vi "Cluster.GetAllContolReferencesRecursive.vi"(6 "error in (no error)":errorcluster, 9 "cluster refnum":refnum<vi>) -> (0 "error out":errorcluster, 1 "labels[]":string[](array[string]), 2 "controls[]":refnum<vi>[](array[refnum]))   [LabVIEW 2019, in "Tools.lvlib"]
doc: "The Get All Control References VI recursively determines control references for all objects on the front panel of another VI. This VI takes a front panel reference input and returns an array of references to all controls on that front panel. This VI returns references to all elements of a cluster, including elements in embedded clusters. This VI also returns the element types of arrays embedded in cluster elements."
uses:
  Tools.lvlib
panel:
  # "Select Help»Show Context Help and move the cursor over the VI icon to display help for this VI."
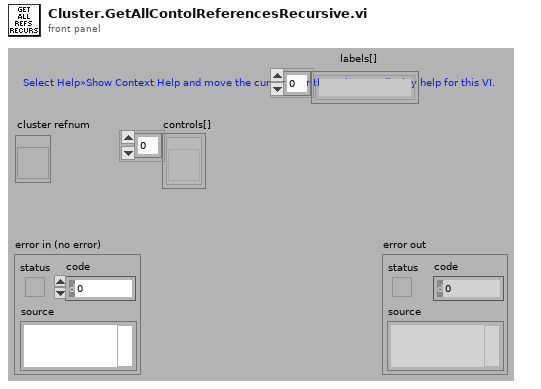
[diagram p1: front panel]
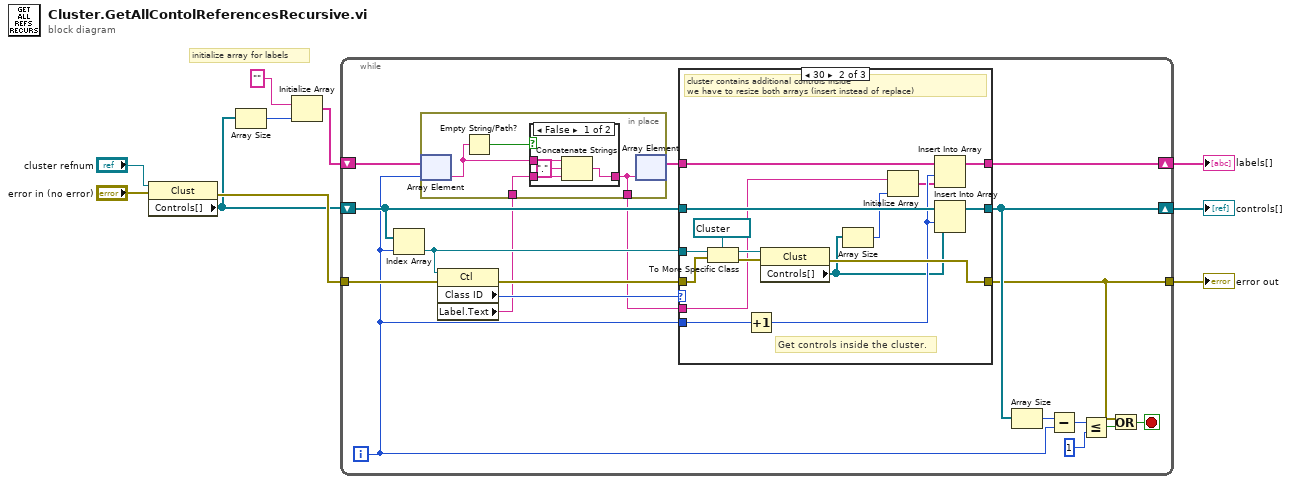
[diagram p0: block diagram]
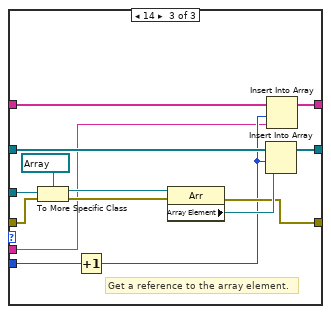
[diagram p4: hidden frame]
diagram:
  # "initialize array for labels"
  n1 = property class="Clust"(reference="cluster refnum", error in="error in (no error)") -> (error out=w8:errorcluster, "Controls[]"=w5:refnum<vi>[])  [unwired: 1 out]
  n2 = Array Size(array=w5) -> (size(s)=w4:i32)
  n3 = Initialize Array("", w4) -> (w3:string[])
  n4 = while {
    shift-right: [w20] -> w10
    shift-left: w5 -> [w21]
    tunnel: w8 -> [w19]
    tunnel: [w11] -> w7
    shift-right: [w17] -> w2
    shift-left: w3 -> [w16]
    i -> [w14]
    stop <- w24 stop-if-true
    n5 = Index Array(array=w21, index=w14) -> (element=w22:refnum<vi>)
    n6 = property class="Ctl"(reference=w22, error in=w19) -> (error out=w18:errorcluster, "Class ID"=w23:u32, "Label.Text"=w13:string)  [unwired: 1 out]
    n7 = in-place {
      in-place-border: w13 -> [w31]
      in-place-border: [w29] -> w12
      n8 = in-place-array #1(w16, w14) -> (w30:string)
      n9 = Empty String/Path?(string/path=w30) -> (empty?=w32:bool)
      n10 = case shown="False" w32 {
        tunnel: w31 -> [w35 w37]
        tunnel: [w34 w37] -> w29
        tunnel: w30 -> [w36 _]
        frame False {
          n11 = Concatenate Strings(w36, "." ("string"), w35) -> (w34:string)
        }
        frame True {
        }
      }
      n12 = in-place-array #1(w29) -> (w15:string[])  [unwired: 1 out]
    }
    n13 = case shown="30" w23 {
      tunnel: w22 -> [_ w56 w70]
      tunnel: w21 -> [w40 w53 w67]
      tunnel: w14 -> [_ w52 w66]
      tunnel: [w40 w48 w61] -> w20
      tunnel: w18 -> [w39 w51 w64]
      tunnel: [w39 w49 w62] -> w11
      tunnel: w15 -> [w38 w47 w60]
      tunnel: [w38 w46 w59] -> w17
      tunnel: w12 -> [_ w44 w57]
      frame Default {
      }
      frame 30 {
        # "Get controls inside the cluster."
        # "cluster contains additional controls inside\nwe have to resize both arrays (insert instead of replace)"
        n14 = To More Specific Class(target class=refnum<vi> refnum, reference=w56, error in=w51) -> (specific class reference=w55:refnum<vi>, error out=w50:errorcluster)
        n15 = Increment(x=w52) -> (x+1=w45:i32)
        n16 = property class="Clust"(reference=w55, error in=w50) -> (error out=w49:errorcluster, "Controls[]"=w42:refnum<vi>[])  [unwired: 1 out]
        n17 = Array Size(array=w42) -> (size(s)=w41:i32)
        n18 = Initialize Array(w44, w41) -> (w43:string[])
        n19 = Insert Into Array(array=w47, index=w45, new element=w43) -> (w46:string[])
        n20 = Insert Into Array(array=w53, index=w45, new element=w42) -> (w48:refnum<vi>[])
      }
      frame 14 {
        # "Get a reference to the array element."
        n21 = To More Specific Class(target class=refnum<vi> refnum ("target class 2"), reference=w70, error in=w64) -> (specific class reference=w69:refnum<vi>, error out=w63:errorcluster)
        n22 = Increment(x=w66) -> (x+1=w58:i32)
        n23 = property class="Arr"(reference=w69, error in=w63) -> (error out=w62:errorcluster, "Array Element"=w65:refnum<vi>)  [unwired: 1 out]
        n24 = Insert Into Array(array=w67, index=w58, new element=w65) -> (w61:refnum<vi>[])
        n25 = Insert Into Array(array=w60, index=w58, new element=w57) -> (w59:string[])
      }
    }
    n26 = Array Size(array=w20) -> (size(s)=w28:i32)
    n27 = Subtract(x=w28, y=w14) -> (x-y=w27:i32)
    n28 = Less Or Equal?(x=w27, y=1) -> (x <= y?=w25:bool)
    n29 = Or(x=w11, y=w25) -> (x .or. y?=w24:bool)
  }
  "controls[]" <- w10
  "error out" <- w7
  "labels[]" <- w2
